vi "Append array.vi"(10 "new section":dbl[](array[numeric]), 11 "Array":dbl[](array[numeric])) -> (3 "Array 2":dbl[](array[numeric]))   [LabVIEW 2018]
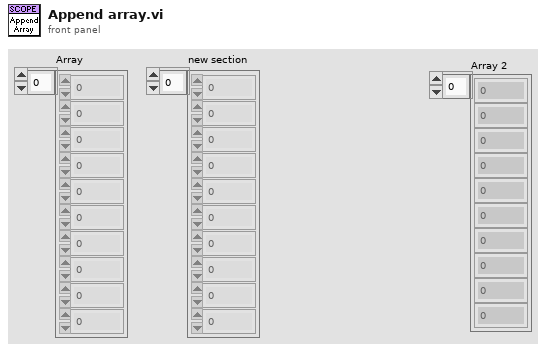
[diagram p1: front panel]
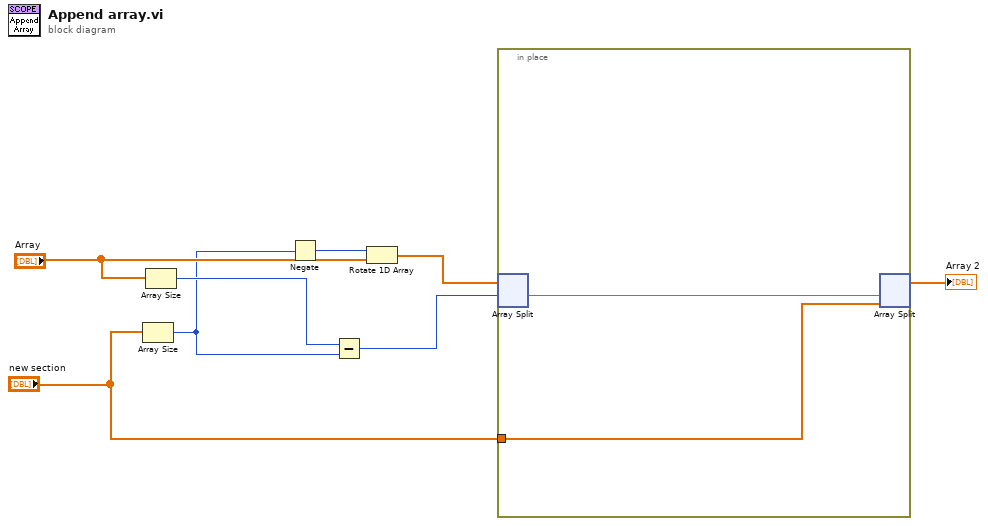
[diagram p0: block diagram]
diagram:
  n1 = Array Size(array="new section") -> (size(s)=w3:i32)
  n2 = Array Size(array="Array") -> (size(s)=w4:i32)
  n3 = Negate(x=w3) -> (-x=w6:i32)
  n4 = Subtract(x=w4, y=w3) -> (x-y=w2:i32)
  n5 = Rotate 1D Array(1:"Array", 2:w6) -> (0:w7:dbl[])
  n6 = in-place {
    in-place-border: "new section" -> [w10]
    n7 = in-place-split #1(w7, w2) -> (w9:dbl[])  [unwired: 1 out]
    n8 = in-place-split #1(w9, w10) -> (→"Array 2":dbl[])  [unwired: 1 out]
  }
